vi "Put Object.vi"(7 "Object Parameters":T1={"Content Type"="binary/octet-stream", "ACL"=enum."private", "Storage Class"=enum."STANDARD", "User-Defined Metadata"=[]}, 8 "error in (no error)":errorcluster, 9 "Object Data":string, 10 "Object Path":string, 11 "Bucket in":refnum<class "Bucket.lvclass">) -> (0 "error out":errorcluster, 3 "Bucket out":refnum<class "Bucket.lvclass">)   [LabVIEW 2015, in "NI_AWS_S3.lvlib" / "Bucket.lvclass"]
doc: "This implementation of the PUT operation adds an object to a bucket. You must have WRITE permissions on a bucket to add an object to it."
uses:
  Bucket.lvclass
  PUT Object Request Parameters.ctl
  ACL.ctl
  Storage Class.ctl
  Core/HTTP Request/Name Value Pair.ctl
  Core/HTTP Request/Request Options.ctl
  Core/HTTP Request/Region handling.ctl
  Core/HTTP Request/URL formatting.ctl
  Bucket.lvclass/Bucket.ctl
  Read Name.vi
  Core/HTTP Request/HTTP Request.lvclass
  Object/Object.lvlib
  NI_AWS_S3.lvlib
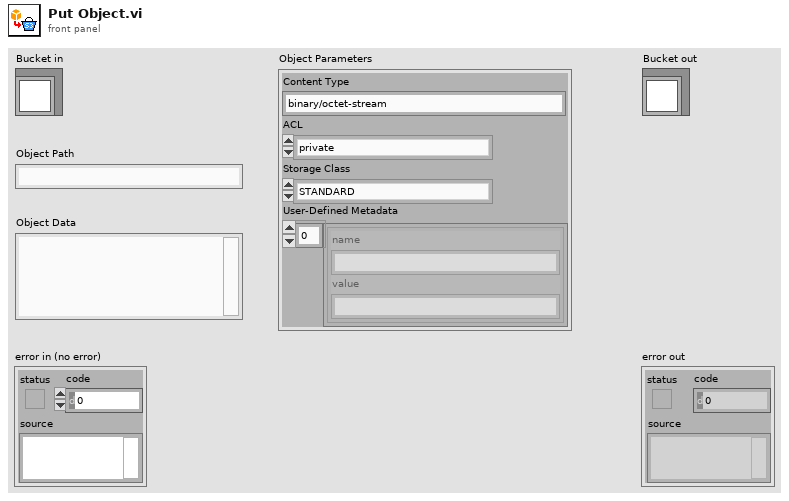
[diagram p1: front panel]
types:
  T1 = typedef "NI_AWS_S3.lvlib/PUT Object Request Parameters.ctl" = cluster{"Content Type":string, "ACL":T2, "Storage Class":T3, "User-Defined Metadata":T4[]}
  T2 = typedef "NI_AWS_S3.lvlib/ACL.ctl" = enum16{"private", "public-read", "public-read-write", "aws-exec-read", "authenticated-read", "bucket-owner-read", "bucket-owner-full-control"}
  T3 = typedef "NI_AWS_S3.lvlib/Storage Class.ctl" = enum16{"STANDARD", "REDUCED_REDUNDANCY"}
  T4 = typedef "NI_AWS_Core.lvlib/HTTP Request.lvclass/Name Value Pair.ctl" = cluster{"name":string, "value":string}
  T5 = typedef "NI_AWS_Core.lvlib/HTTP Request.lvclass/Region handling.ctl" = enum16{"use region everywhere", "use region (authentication only)", "use region (URL only)", "ignore region everwhere"}
  T6 = typedef "NI_AWS_Core.lvlib/HTTP Request.lvclass/Request Options.ctl" = cluster{"request headers":T4[], "request parameters":T4[], "request body":string, "region handling":T5, "URL formatting":T7}
  T7 = typedef "NI_AWS_Core.lvlib/HTTP Request.lvclass/URL formatting.ctl" = enum16{"region-", "region."}
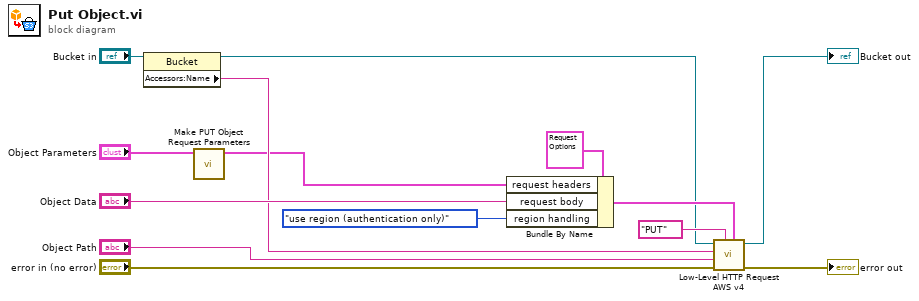
[diagram p0: block diagram]
diagram:
  n1 = property class="Bucket"(reference="Bucket in") -> (reference out=w3:refnum<class "Bucket.lvclass">, "Accessors:Name"=w9:string)  [unwired: 1 in, 1 out]
  n2 = call "Make PUT Object Request Parameters.vi"("PUT Object Request Parameters"="Object Parameters") -> ("HTTP Headers"=w7:T4[])  [unwired: 10 in]
  n3 = Bundle By Name(cluster=T6 {"request headers"=[], "request parameters"=[], "request body"="", "region handling"=enum."use region everywhere", "URL formatting"=enum."region."} ("Request Options"), "request headers"=w7, "request body"="Object Data", "region handling"=Region_handling."use region (authentication only)") -> (w5:T6)
  n4 = call "Low-Level HTTP Request AWS v4.vi"("Request Options"=w5, "HTTP-Verb"="PUT", "error in (no error)"="error in (no error)", "URL Suffix"="Object Path", "URL Prefix"=w9, "AWS Core in"=w3) -> ("error out"=→"error out":errorcluster, "AWS Core out"=→"Bucket out":refnum<class "Bucket.lvclass">)  [unwired: 2 in, 2 out]
